vi "PR4000 setpoint.vi"(1 "new setpoint":dbl=2500.0, 2 "Channel":i16=1) -> ()   [LabVIEW 2019]
uses:
  MKS_PR4000/PR4000_driver/serial_settings.ctl
  MKS_PR4000/PR4000_driver/MKS_PR4000.lvclass
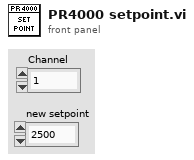
[diagram p1: front panel]
types:
  T1 = typedef "MKS_PR4000.lvlib/MKS_PR4000.lvclass/serial_settings.ctl" = cluster{"Baud Rate (9600)":u32, "Serial Settings:Parity (Odd)":u16, "Serial Settings:Data Bits (7)":u16}
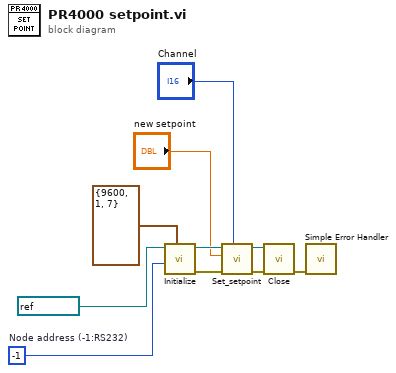
[diagram p0: block diagram]
diagram:
  w9 = i8 -1  # Node address (-1:RS232)
  n1 = call "Initialize.vi"("Serial settings"=T1 {"Baud Rate (9600)"=9600, "Serial Settings:Parity (Odd)"=1, "Serial Settings:Data Bits (7)"=7}, "Node address (-1:RS232)"=w9, "VISA resource name"=refnum<visa-resource-name> "COM5" ("VISA resources")) -> ("error out"=w8:errorcluster, "MKS_PR4000 out"=w7:refnum<class "MKS_PR4000.lvclass">)  [unwired: 7 in]
  n2 = call "Set_setpoint.vi"("Channel"="Channel", "error in (no error)"=w8, "new setpoint"="new setpoint", "MKS_PR4000 in"=w7) -> ("error out"=w5:errorcluster, "MKS_PR4000 out"=w6:refnum<class "MKS_PR4000.lvclass">)  [unwired: 6 in]
  n3 = call "Close.vi"("error in (no error)"=w5, "MKS_PR4000 in"=w6) -> ("error out"=w10:errorcluster)  [unwired: 8 in, 1 out]
  n4 = call <vilib>:"Simple Error Handler.vi"("error in (no error)"=w10) -> ()  [unwired: 4 in, 5 out]
